vi "MKS670_GPIB_calib.vi"(5 "ref_msg":refnum<vi>, 7 "wait":i32=30, 8 "error in":errorcluster, 11 "GPIB in":string) -> (0 "error out":errorcluster, 3 "GPIB out":string, 4 "status":bool)   [LabVIEW 2019]
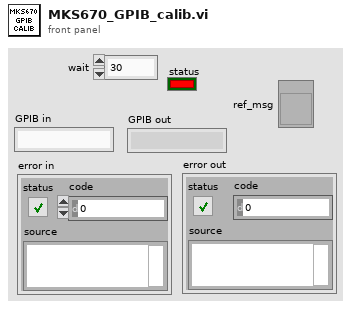
[diagram p1: front panel]
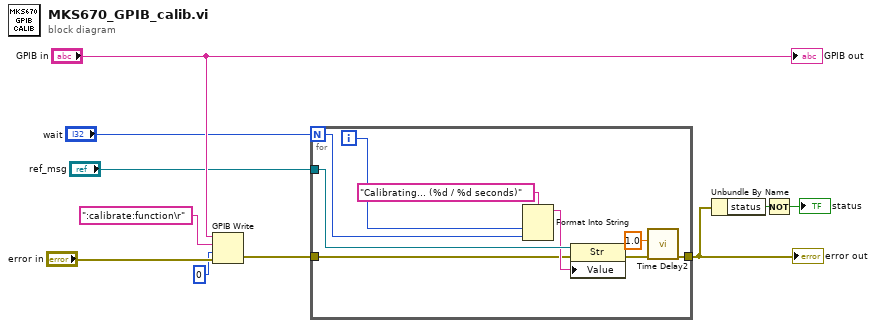
[diagram p0: block diagram]
diagram:
  n1 = GPIB Write(0:"GPIB in", 1:":calibrate:function\r" ("data"), 2:i16 0 ("mode (0)"), 3:"error in") -> (6:w2:errorcluster)  [unwired: 1 in, 1 out]
  n2 = for {
    N: "wait" -> [w17]
    tunnel: "ref_msg" -> [w16]
    tunnel: w2 -> [w13]
    tunnel: [w11] -> w1
    i -> [w19]
    n3 = Format Into String(format string="Calibrating... (%d / %d seconds)", w19, w17) -> (resulting string=w15:string)  [unwired: 2 in, 1 out]
    n4 = property class="Str"(reference=w16, error in=w13, "Value"=w15) -> (error out=w12:errorcluster)  [unwired: 1 out]
    n5 = call "Time Delay2"("error in (no error)"=w12, "Delay Time (s)"=1.0) -> ("error out"=w11:errorcluster)  [unwired: 9 in]
  }
  "error out" <- w1
  n6 = Unbundle By Name(w1) -> ("status"=w9:bool)
  n7 = Not(x=w9) -> (.not. x?=→"status":bool)
  "GPIB out" <- "GPIB in"
